vi "Format Item Names.vi"(5 "Displayed Indices":i32[](array[numeric]), 7 "Abbreviate Names?":bool, 9 "Saved VI Data":T1, 11 "New VI Data":T1) -> (0 "Number of Modified Items":i32, 2 "Item Names":string[](array[string]))   [LabVIEW 2023, in "VI Properties Editor.lvlib"]
doc: "Formats the VI names into item names to be displayed in the main listbox, based on <B>Abbreviate Names?</B> and if modifications have been made."
uses:
  VI Properties Editor.lvlib
  <vilib>/picture/picture.llb/imagedata.ctl
  CTLs/VI Properties.ctl
  CTLs/Control Properties.ctl
  CTLs/VI Data Map.ctl
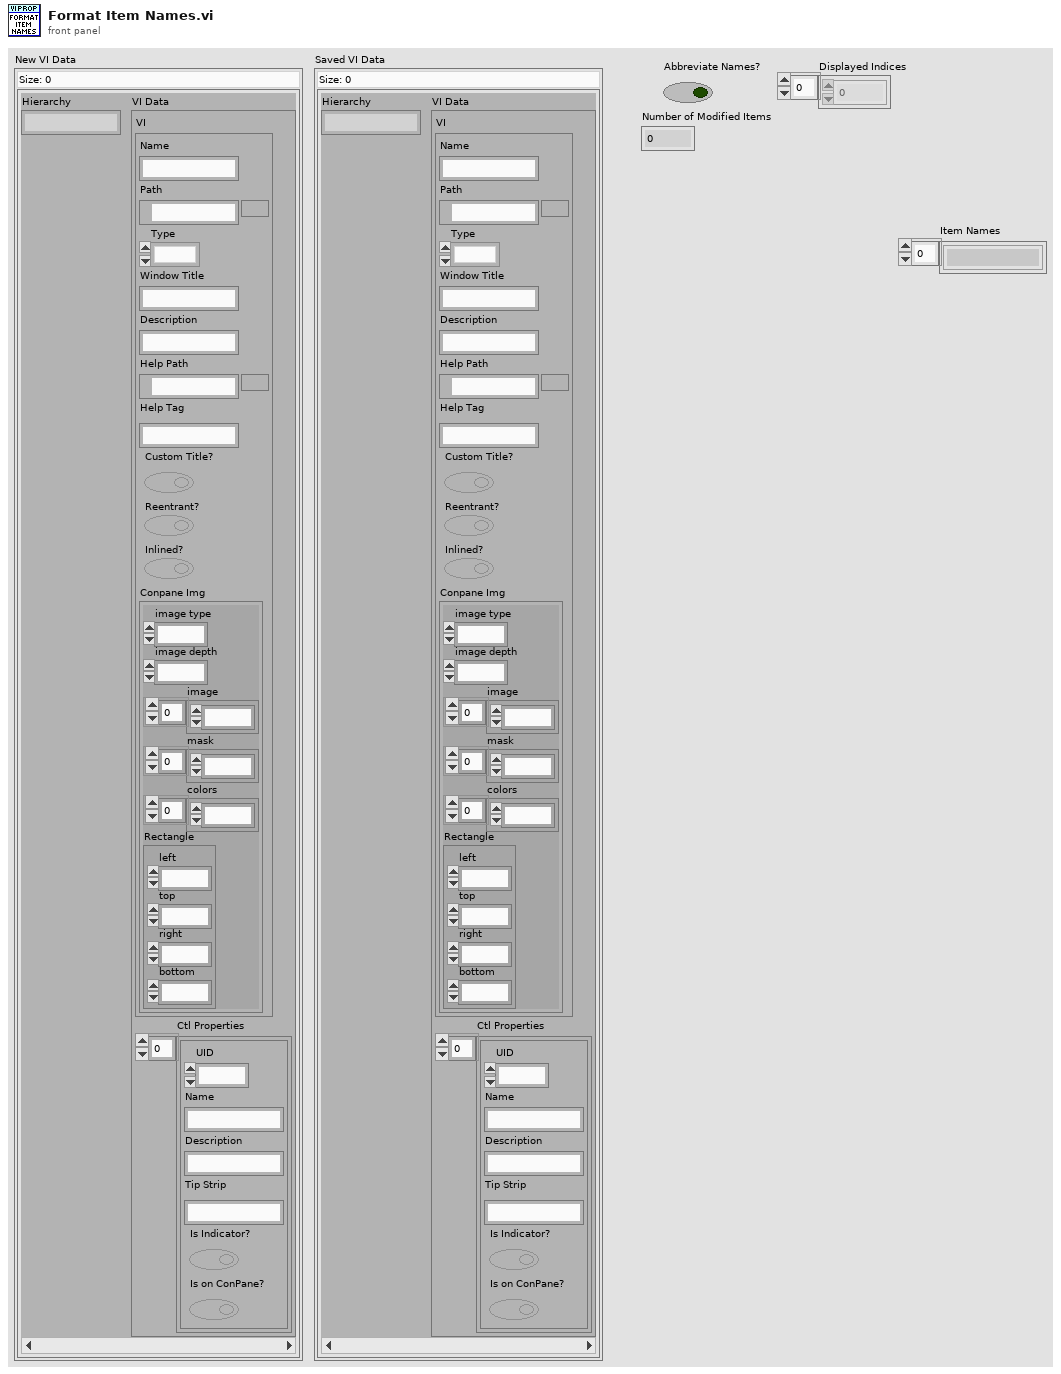
[diagram p1: front panel]
types:
  T1 = typedef "VI Properties Editor.lvlib/VI Data Map.ctl" = map{string, cluster{"VI":T2, "Ctl Properties":T4[]}}
  T2 = typedef "VI Properties Editor.lvlib/VI Properties.ctl" = cluster{"Name":string, "Path":path, "Type":enum32{"invalid VI type", "Standard VI", "Control VI", "Global VI", "Polymorphic VI", "Configuration VI", "SubSystem", "Facade VI", "Method VI", "Statechart Diagram VI"}, "Window Title":string, "Description":string, "Help Path":path, "Help Tag":string, "Custom Title?":bool, "Reentrant?":bool, "Inlined?":bool, "Conpane Img":T3}
  T3 = typedef "imagedata.ctl" = cluster{"image type":i32, "image depth":i32, "image":u8[], "mask":u8[], "colors":u32[], "Rectangle":cluster{"left":i16, "top":i16, "right":i16, "bottom":i16}}
  T4 = typedef "VI Properties Editor.lvlib/Control Properties.ctl" = cluster{"UID":i32, "Name":string, "Description":string, "Tip Strip":string, "Is Indicator?":bool, "Is on ConPane?":bool}
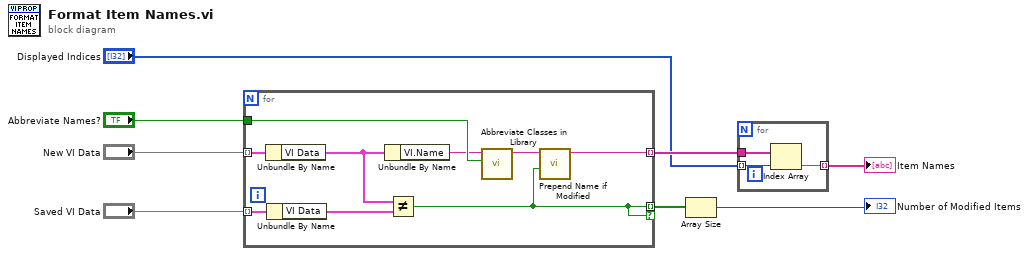
[diagram p0: block diagram]
diagram:
  n1 = for {
    tunnel: "Saved VI Data" -> [w17] mode=indexing
    tunnel: "New VI Data" -> [w13] mode=indexing
    tunnel: "Abbreviate Names?" -> [w16]
    tunnel: [w15] -> w6 mode=indexing
    tunnel: [w14] -> w3 mode=indexing if=w14
    n2 = Unbundle By Name(w13) -> ("VI Data"=w9:cluster{"VI":T2, "Ctl Properties":T4[]})
    n3 = Unbundle By Name(w17) -> ("VI Data"=w10:cluster{"VI":T2, "Ctl Properties":T4[]})
    n4 = Unbundle By Name(w9) -> ("VI.Name"=w12:string)
    n5 = Not Equal?(x=w9, y=w10) -> (x != y?=w14:bool)
    n6 = call "Abbreviate Classes in Library.vi"("Abbreviate Name?"=w16, "Name"=w12) -> ("Name out"=w11:string)  [unwired: 9 in]
    n7 = call "Prepend Name if Modified.vi"("Modified?"=w14, "VI Name"=w11) -> ("VI Name out"=w15:string)  [unwired: 9 in]
  }
  n8 = Array Size(array=w3) -> (size(s)=→"Number of Modified Items":i32)
  n9 = for {
    tunnel: w6 -> [w20]
    tunnel: "Displayed Indices" -> [w19] mode=indexing
    tunnel: [w18] -> w5 mode=indexing
    n10 = Index Array(array=w20, index=w19) -> (element=w18:string)
  }
  "Item Names" <- w5
